vi "read.vi"() -> ()   [LabVIEW 2024]
uses:
  <vilib>/Utility/NIReport.llb/Report Type.ctl
  <vilib>/addons/_office/excel.llb/Excel Get Data ([str]).vi
  <vilib>/Utility/NIReport.llb/NI_report.lvclass
  <vilib>/Utility/NIReport.llb/Excel/NI_Excel.lvclass
  <vilib>/Utility/NIReport.llb/NI_ReportGenerationCore.lvlib
  <vilib>/addons/_office/NI_ReportGenerationToolkit.lvlib
panel:
  out "实验时间（s）":i32
  in  "表":i32
  out "错误输出":errorcluster
  out "Q":string
  out "p":string
  out "T":string
  in  "end (-1, -1)":cluster{"row":i32, "column":i32}={"row"=-1, "column"=-1}
  in  "start (-1, -1)":cluster{"row":i32, "column":i32}={"row"=-1, "column"=-1}
  out "sheet 数量":i32
  out "data":string[][](array[string])
  in  "读取数据":bool
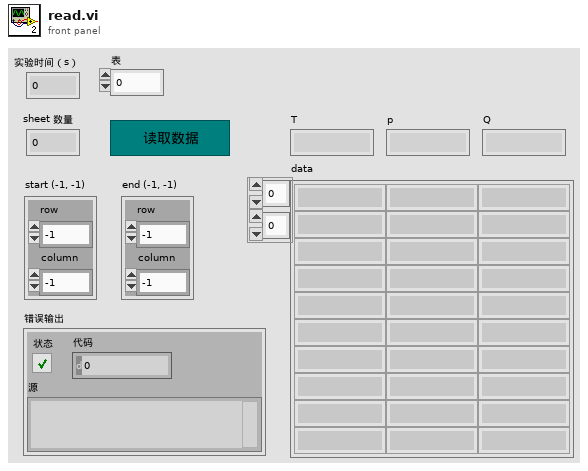
[diagram p1: front panel]
types:
  T1 = typedef "NI_ReportGenerationCore.lvlib/Report Type.ctl" = enum16{"HTML", "Word", "Excel"}
  T2 = enum16{"maximized", "minimized", "normal", "no change"}
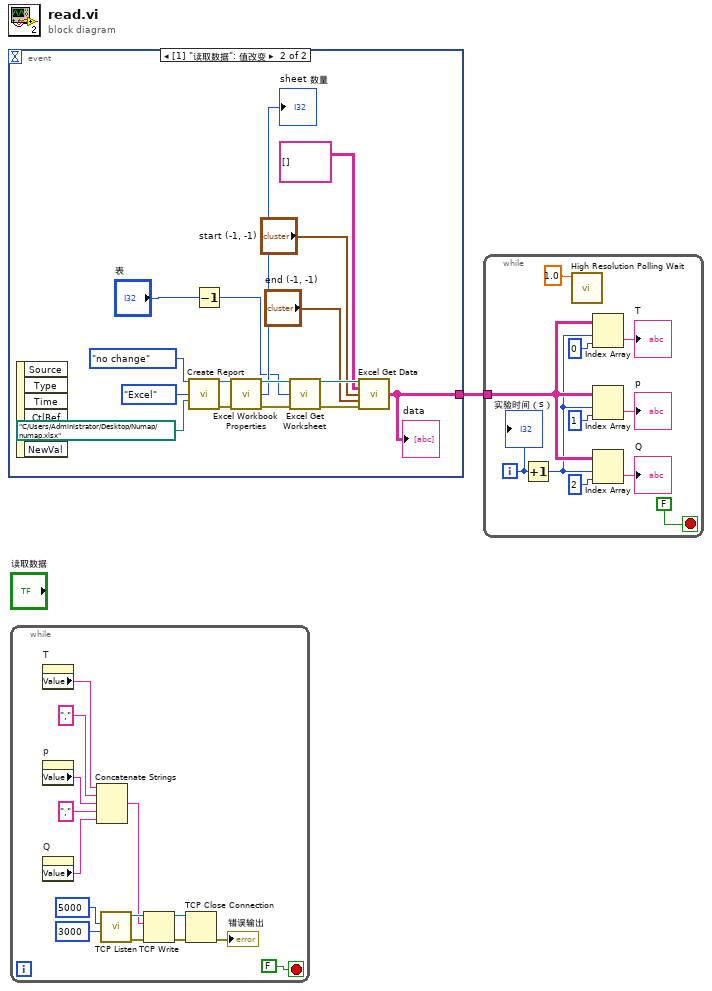
[diagram p0: block diagram]
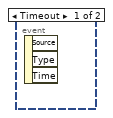
[diagram p2: hidden frame]
diagram:
  n1 = event shown="[1] \"读取数据\": 值改变" {
    selector: _ -> [_ _]
    dyn-events: _ -> [_ _]
    timeout: _ -> [_ _]
    tunnel: [_ w4] -> w1
    event Timeout {
      n2 = event-data() -> ()  [unwired: 1 in, 3 out]
    }
    event "读取数据": Value Change {
      n3 = event-data() -> ()  [unwired: 1 in, 6 out]
      n4 = call <vilib>:"Create Report.vi"("window state (normal)"=T2."no change", "report type"=Report_Type."Excel", "template (empty)"=path "C:/Users/Administrator/Desktop/Numap/numap.xlsx") -> ("report out"=w13:refnum<class "NI_report.lvclass">, "error out"=w11:errorcluster)  [unwired: 11 in]
      n5 = Decrement(x="表") -> (x-1=w2:i32)
      n6 = call <vilib>:"Excel Workbook Properties.vi"("report in"=w13, "error in (no error)"=w11) -> ("report out"=w12:refnum<class "NI_report.lvclass">, "worksheets count"=→"sheet 数量":i32, "error out"=w10:errorcluster)  [unwired: 10 in, 1 out]
      n7 = call <vilib>:"Excel Get Worksheet.vi"("report in"=w12, "worksheet index (0)"=w2, "error in (no error)"=w10) -> ("report out"=w15:refnum<class "NI_report.lvclass">, "error out"=w9:errorcluster)  [unwired: 11 in]
      n8 = call-poly <vilib>:"Excel Get Data.vi"("report in"=w15, "data type"=string[][] [], "start (-1, -1)"="start (-1, -1)", "end (-1, -1)"="end (-1, -1)", "error in (no error)"=w9) -> ("data"=w4:string[][])  [unwired: 8 in, 2 out]
      "data" <- w4
    }
  }
  n9 = while {
    stop <- FALSE stop-if-true
    n10 = property on="T" class="Str"() -> ("Value"=w20:string)  [unwired: 2 in, 2 out]
    n11 = property on="p" class="Str"() -> ("Value"=w19:string)  [unwired: 2 in, 2 out]
    n12 = property on="Q" class="Str"() -> ("Value"=w18:string)  [unwired: 2 in, 2 out]
    n13 = Concatenate Strings(w20, "," ("字符串"), w19, "," ("字符串"), w18) -> (w22:string)
    n14 = call <vilib>:"TCP Listen.vi"("timeout ms (wait forever: -1)"=3000, "port"=u16 5000) -> ("error out"=w28:errorcluster, "connection ID"=w27:refnum<k5>)  [unwired: 5 in, 3 out]
    n15 = TCP Write(connection ID=w27, data in=w22, error in (no error)=w28) -> (connection ID out=w26:refnum<k5>, error out=w30:errorcluster)  [unwired: 1 in, 1 out]
    n16 = TCP Close Connection(connection ID=w26, error in (no error)=w30) -> (error out=→"错误输出":errorcluster)  [unwired: 1 in, 1 out]
  }
  n17 = while {
    tunnel: w1 -> [w34]
    i -> [w39]
    stop <- FALSE stop-if-true
    n18 = Increment(x=w39) -> (x+1=w33:i32)
    n19 = call <vilib>:"High Resolution Polling Wait.vi"("seconds to wait"=1.0) -> ()  [unwired: 10 in, 1 out]
    n20 = Index Array(array=w34, index (row)=w33, index (col)=0 ("禁用的索引 (列)")) -> (element=→"T":string)
    n21 = Index Array(array=w34, index (row)=w33, index (col)=1 ("禁用的索引 (列)")) -> (element=→"p":string)
    n22 = Index Array(array=w34, index (row)=w33, index (col)=2 ("禁用的索引 (列)")) -> (element=→"Q":string)
    "实验时间（s）" <- w39
  }
